vi "READ Serial.vi"(5 "error in":errorcluster, 8 "VISA Resource Name In":refnum<visa-resource-name>="COM2") -> (1 "error out":errorcluster, 2 "VISA Resource Name Out":refnum<visa-resource-name>, 3 "Output String":string)   [LabVIEW 2013]
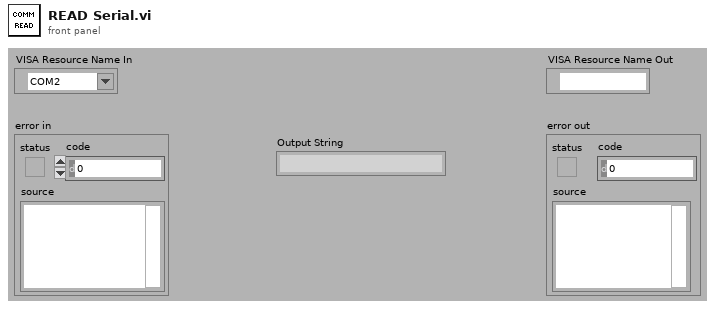
[diagram p1: front panel]
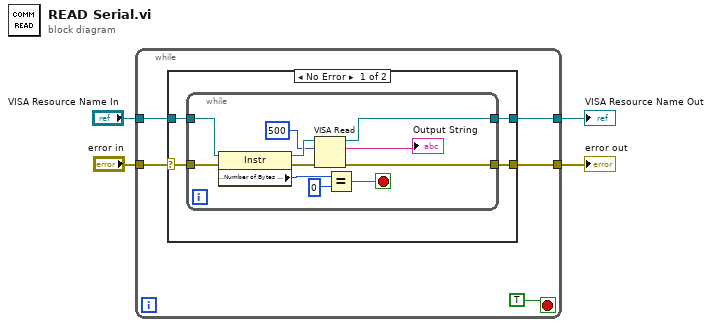
[diagram p0: block diagram]
diagram:
  n1 = while {
    tunnel: "error in" -> [w5]
    tunnel: "VISA Resource Name In" -> [w9]
    tunnel: [w7] -> w2
    tunnel: [w6] -> w1
    stop <- TRUE stop-if-true
    n2 = case shown="No Error" w5 {
      selector: w5 -> [w10 w26]
      tunnel: w9 -> [w11 w25]
      tunnel: [w12 w26] -> w7
      tunnel: [w13 w25] -> w6
      frame No Error {
        n3 = while {
          tunnel: [w21] -> w13
          tunnel: [w20] -> w12
          tunnel: w11 -> [w16]
          tunnel: w10 -> [w15]
          stop <- w18 stop-if-true
          n4 = property class="Instr"(reference=w16, error in=w15) -> (reference out=w22:refnum<visa-resource-name>, error out=w19:errorcluster, "Serial Settings:Number of Bytes at Serial Port"=w24:u32)
          n5 = VISA Read(VISA resource name=w22, byte count=u32 500, error in (no error)=w19) -> (VISA resource name out=w21:refnum<visa-resource-name>, read buffer=→"Output String":string, error out=w20:errorcluster)  [unwired: 1 out]
          n6 = Equal?(x=w24, y=u32 0) -> (x = y?=w18:bool)
        }
      }
      frame Error {
      }
    }
  }
  "error out" <- w2
  "VISA Resource Name Out" <- w1
